vi "Sort Complex Numbers (Magnitude, obs).vi"(10 "Order":enum16{"Ascending", "Descending"}(ring), 11 "Complex Numbers":cdb[](array[numeric]) format="%#.6g") -> (0 "error":i32, 2 "Sorted Index":i32[](array[numeric]), 3 "Sorted Complex Numbers":cdb[](array[numeric]) format="%#.6g")   [LabVIEW 2014, in "NI_AALPro.lvlib"]
uses:
  NI_AALPro.lvlib
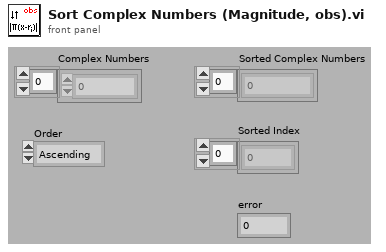
[diagram p1: front panel]
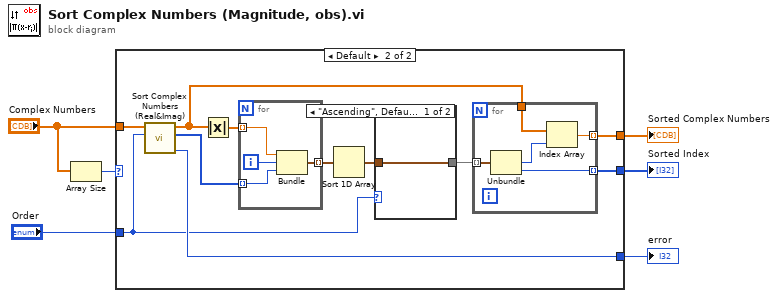
[diagram p0: block diagram]
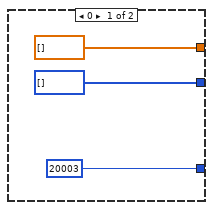
[diagram p2: hidden frame]
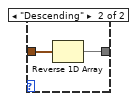
[diagram p3: hidden frame]
diagram:
  n1 = Array Size(array="Complex Numbers") -> (size(s)=w3:i32)
  n2 = case shown="Default" w3 {
    tunnel: "Complex Numbers" -> [_ w12]
    tunnel: [i32[] [] w18] -> w6
    tunnel: [cdb[] [] ("CDB") w17] -> w5
    tunnel: "Order" -> [_ w13]
    tunnel: [20003 ("empty array") w14] -> w1
    frame 0 {
    }
    frame Default {
      n3 = call "Sort Complex Numbers (Real&Imag).vi"("Order"=w13, "Complex Numbers"=w12) -> ("error"=w14:i32, "Sorted Index"=w10:i32[], "Sorted Complex Numbers"=w11:cdb[])  [unwired: 7 in]
      n4 = Absolute Value(x=w11) -> (abs(x)=w20:dbl[])
      n5 = for {
        tunnel: [w31] -> w19 mode=indexing
        tunnel: w20 -> [w32] mode=indexing
        tunnel: w10 -> [w29] mode=indexing
        i -> [w30]
        n6 = Bundle("Numeric"=w32, w30, "Numeric"=w29) -> (w31:cluster{"Numeric":dbl, i32, "Numeric":i32})  [unwired: 1 in]
      }
      n7 = Sort 1D Array(array=w19) -> (sorted array=w16:cluster{"Numeric":dbl, i32, "Numeric":i32}[])
      n8 = case shown="\"Ascending\", Default" w13 {
        tunnel: w16 -> [w21 w23]
        tunnel: [w21 w22] -> w15
        frame "Ascending", Default {
        }
        frame "Descending" {
          n9 = Reverse 1D Array(array=w23) -> (reversed array=w22:cluster{"Numeric":dbl, i32, "Numeric":i32}[])
        }
      }
      n10 = for {
        tunnel: w15 -> [w28] mode=indexing
        tunnel: w11 -> [w27]
        tunnel: [w26] -> w17 mode=indexing
        tunnel: [w24] -> w18 mode=indexing
        n11 = Unbundle(w28) -> (w25:i32, "Numeric"=w24:i32)  [unwired: 1 out]
        n12 = Index Array(array=w27, index=w25) -> (element=w26:cdb)
      }
    }
  }
  "Sorted Index" <- w6
  "Sorted Complex Numbers" <- w5
  "error" <- w1
